vi "Create Container.vi"(8 "Error In":errorcluster, 11 "Tab Widget Builder in":refnum<class "Tab Widget Builder.lvclass">) -> (0 "Error Out":errorcluster, 2 "Container":refnum<class "QWidget.lvclass">, 3 "Tab Widget Builder out":refnum<class "Tab Widget Builder.lvclass">)   [LabVIEW 2013, in "Tab Widget Builder.lvclass"]
uses:
  Tab Widget Builder.lvclass
  src/LabVIEW/Qt Widgets/QWidget/QWidget.lvclass
  src/LabVIEW/Qt Widgets/QTabWidget/QTabWidget.lvclass
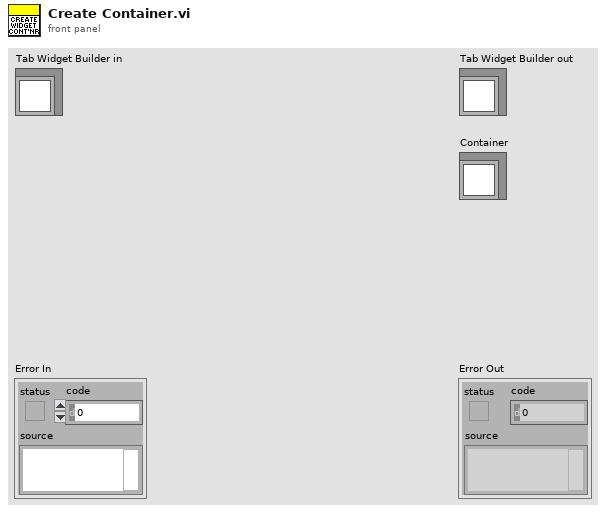
[diagram p1: front panel]
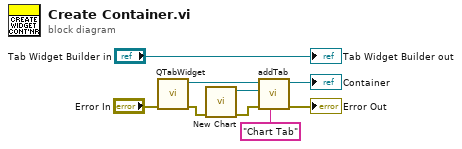
[diagram p0: block diagram]
diagram:
  n1 = call "QTabWidget.vi"("Error In"="Error In") -> ("Error Out"=w3:errorcluster, "New QTabWidget"=w5:refnum<class "QTabWidget.lvclass">)  [unwired: 9 in]
  n2 = call "New Chart.vi"("Error In"=w3) -> ("Error Out"=w2:errorcluster, "New LQChart"=w6:refnum<class "LQChart.lvclass">)  [unwired: 9 in]
  n3 = call "addTab.vi"("label"="Chart Tab", "Error In"=w2, "widget"=w6, "QTabWidget In"=w5) -> ("Error Out"=→"Error Out":errorcluster, "QTabWidget Out"=→"Container":refnum<class "QTabWidget.lvclass">)  [unwired: 5 in, 1 out]
  "Tab Widget Builder out" <- "Tab Widget Builder in"
